vi "CFTS-Password Dialog.vi"(2 "Parent VI":refnum<vi>) -> (8 "hash":string)   [LabVIEW 2020]
uses:
  <vilib>/security/Message Digest/API/Instances/Byte Array/SHA-256 Byte Array Checksum.vi
  <vilib>/security/Message Digest/API/NI_Message Digest API.lvlib
panel:
  in  "Enter password":string
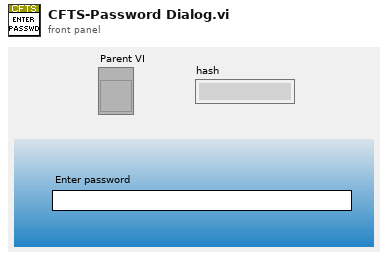
[diagram p1: front panel]
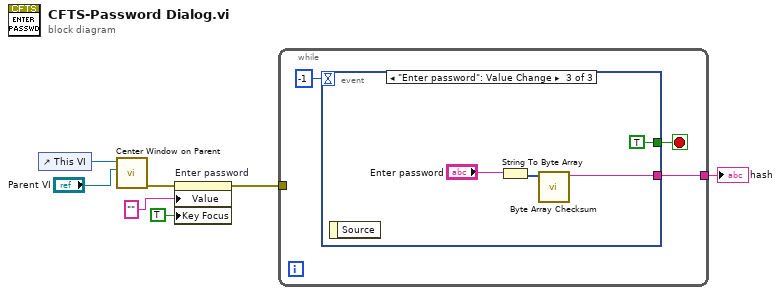
[diagram p0: block diagram]
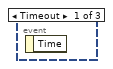
[diagram p2: hidden frame]
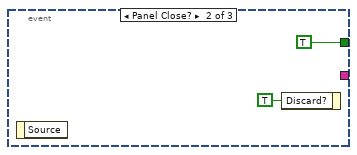
[diagram p3: hidden frame]
diagram:
  n1 = control-ref of="This VI"() -> (w6:refnum<vi>)
  n2 = call "Center Window on Parent.vi"("Parent VI"="Parent VI", "VI in"=w6) -> ("error out"=w4:errorcluster)  [unwired: 8 in, 1 out]
  n3 = property on="Enter password" class="Str"(error in=w4, "Value"="" ("Enter password"), "Key Focus"=TRUE) -> (error out=w3:errorcluster)  [unwired: 1 in, 1 out]
  n4 = while {
    tunnel: [w8] -> w7
    tunnel: w3 -> [_]
    stop <- w9 stop-if-true
    n5 = event shown="[2] \"Enter password\": Value Change" {
      selector: _ -> [_ _ _]
      dyn-events: _ -> [_ _ _]
      timeout: -1 -> [_ _ _]
      tunnel: [_ TRUE TRUE] -> w9
      tunnel: [_ _ w13] -> w8
      event Timeout {
        n6 = event-data() -> ()  [unwired: 1 in, 1 out]
      }
      event Panel Close? {
        n7 = event-data() -> ()  [unwired: 1 in, 1 out]
        n8 = event-data("Discard?"=TRUE) -> ()  [unwired: 1 in, 1 out]
      }
      event "Enter password": Value Change {
        n9 = event-data() -> ()  [unwired: 1 in, 1 out]
        n10 = String To Byte Array(string="Enter password") -> (unsigned byte array=w15:u8[])
        n11 = call-poly <vilib>:"Byte Array Checksum.vi"("buffer"=w15) -> ("digest"=w13:string)  [unwired: 10 in]
      }
    }
  }
  "hash" <- w7
